vi "Ref_3_ch_11-20.vi"(0 "Trip  Ch 11":refnum<vi>, 1 "Trip  Ch 12":refnum<vi>, 3 "Trip  Ch 13":refnum<vi>, 4 "Trip  Ch 14":refnum<vi>, 5 "Trip  Ch 15":refnum<vi>, 7 "Trip  Ch 16":refnum<vi>, 8 "Trip  Ch 17":refnum<vi>, 9 "Trip  Ch 18":refnum<vi>, 10 "Init_F":bool=TRUE, 12 "Trip  Ch 19":refnum<vi>, 13 "Trip  Ch 20":refnum<vi>) -> (14 "Trip  Ch 11 out":refnum<vi>, 15 "Trip  Ch 12 out":refnum<vi>, 16 "Trip  Ch 13 out":refnum<vi>, 17 "Trip  Ch 14 out":refnum<vi>, 19 "Trip  Ch 15 out":refnum<vi>, 20 "Trip  Ch 16 out":refnum<vi>, 21 "Trip  Ch 17 out":refnum<vi>, 23 "Trip  Ch 18 out":refnum<vi>, 24 "Trip  Ch 19 out":refnum<vi>, 25 "Trip  Ch 20 out":refnum<vi>)   [LabVIEW 2017]
panel:
  out "error out":errorcluster
  in  "error in":errorcluster
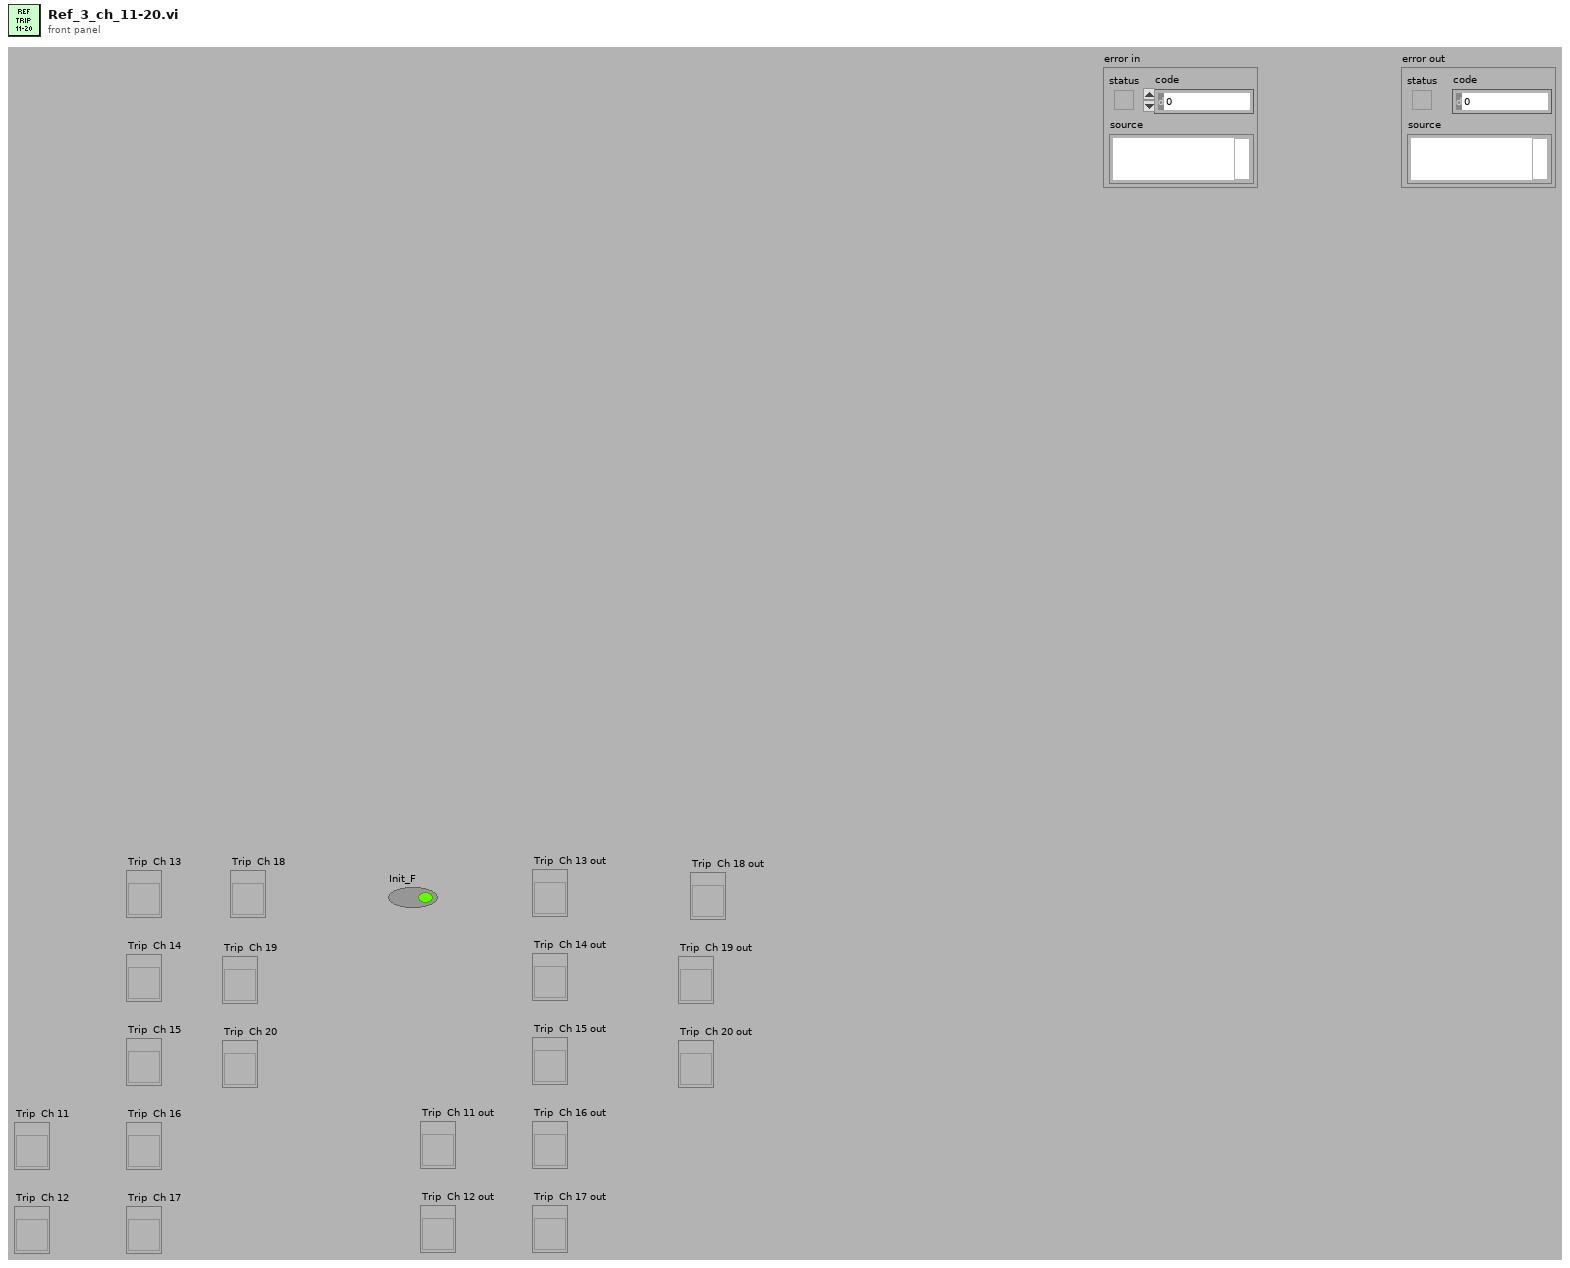
[diagram p1: front panel]
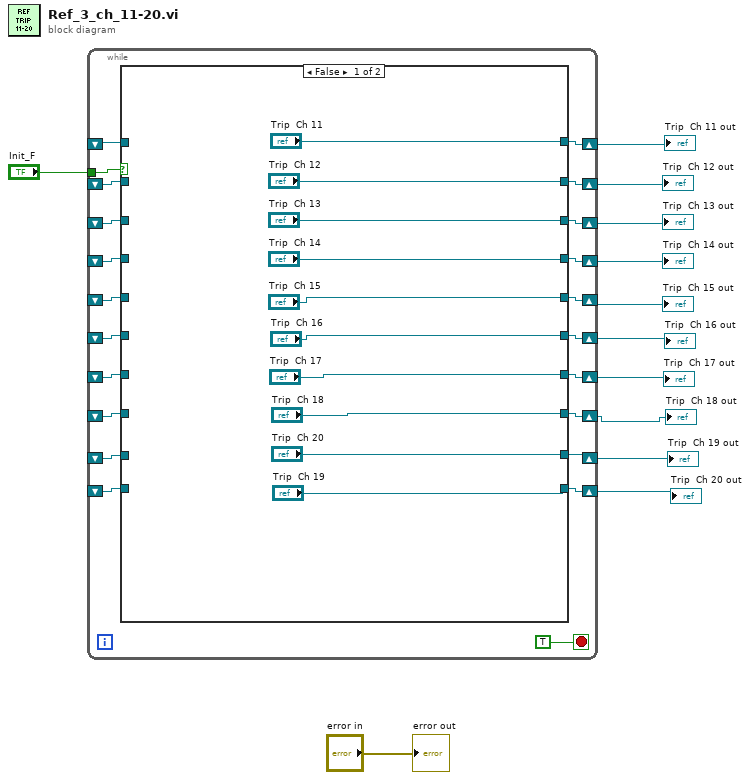
[diagram p0: block diagram]
diagram:
  n1 = while {
    shift-right: [w33] -> w4
    shift-left: _ -> [w32]
    tunnel: "Init_F" -> [w31]
    shift-right: [w30] -> w5
    shift-left: _ -> [w23]
    shift-right: [w29] -> w6
    shift-left: _ -> [w22]
    shift-right: [w28] -> w7
    shift-left: _ -> [w17]
    shift-right: [w27] -> w8
    shift-left: _ -> [w21]
    shift-right: [w26] -> w9
    shift-left: _ -> [w20]
    shift-right: [w25] -> w10
    shift-left: _ -> [w19]
    shift-right: [w24] -> w1
    shift-left: _ -> [w18]
    shift-right: [w16] -> w3
    shift-left: _ -> [w14]
    shift-right: [w15] -> w2
    shift-left: _ -> [w13]
    stop <- TRUE stop-if-true
    n2 = case shown="False" w31 {
      tunnel: ["Trip  Ch 11" w54] -> w33
      tunnel: w32 -> [_ w54]
      tunnel: ["Trip  Ch 12" w47] -> w30
      tunnel: ["Trip  Ch 13" w48] -> w29
      tunnel: ["Trip  Ch 14" w49] -> w28
      tunnel: ["Trip  Ch 15" w50] -> w27
      tunnel: ["Trip  Ch 16" w51] -> w26
      tunnel: ["Trip  Ch 17" w52] -> w25
      tunnel: ["Trip  Ch 18" w53] -> w24
      tunnel: w23 -> [_ w47]
      tunnel: w22 -> [_ w48]
      tunnel: w21 -> [_ w50]
      tunnel: w20 -> [_ w51]
      tunnel: w19 -> [_ w52]
      tunnel: w18 -> [_ w53]
      tunnel: w17 -> [_ w49]
      tunnel: ["Trip  Ch 20" w46] -> w16
      tunnel: ["Trip  Ch 19" w45] -> w15
      tunnel: w14 -> [_ w46]
      tunnel: w13 -> [_ w45]
      frame False {
      }
      frame True {
      }
    }
  }
  "Trip  Ch 18 out" <- w1
  "Trip  Ch 17 out" <- w10
  "Trip  Ch 16 out" <- w9
  "Trip  Ch 15 out" <- w8
  "Trip  Ch 14 out" <- w7
  "Trip  Ch 13 out" <- w6
  "Trip  Ch 12 out" <- w5
  "Trip  Ch 11 out" <- w4
  "Trip  Ch 19 out" <- w3
  "Trip  Ch 20 out" <- w2
  "error out" <- "error in"
